vi "Build Payload.vi"(9 "DO_Port":u64, 11 "Payload In":u64[](array[numeric]) format="%x") -> (3 "Payload Out":u64[](array[numeric]) format="%x")   [LabVIEW 2025]
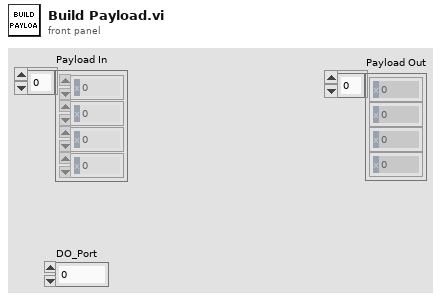
[diagram p1: front panel]
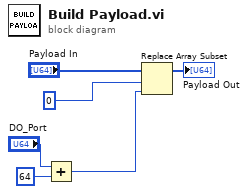
[diagram p0: block diagram]
diagram:
  n1 = Add(x="DO_Port", y=u64 64) -> (x+y=w2:u64)
  n2 = Replace Array Subset(array="Payload In", new element=w2, index=u64 0 ("Index")) -> (→"Payload Out":u64[])
